vi "Manual Control - Connected Device Measurement.vi"(8 "error in":errorcluster, 10 "DER_Measurement":T1, 11 "Master Controller in":refnum<class "EMS User Interface.lvclass">) -> (0 "error out":errorcluster, 3 "Master Controller out":refnum<class "EMS User Interface.lvclass">)   [LabVIEW 2018, in "EMS User Interface Actor.lvlib" / "EMS User Interface.lvclass"]
uses:
  EMS User Interface.lvclass
  <vilib>/ORNL/CSEISMIC DDS/CSEISMIC DDS Base/Data Types/DER_Measurement.ctl
  <vilib>/ORNL/CSEISMIC DDS/CSEISMIC DDS Base/Data Types/Controls/DeviceID.ctl
  EMS User Interface.lvclass/EMS User Interface.ctl
  <vilib>/ORNL/CSEISMIC DDS/CSEISMIC DDS Base/CSEISMIC DDS.lvclass
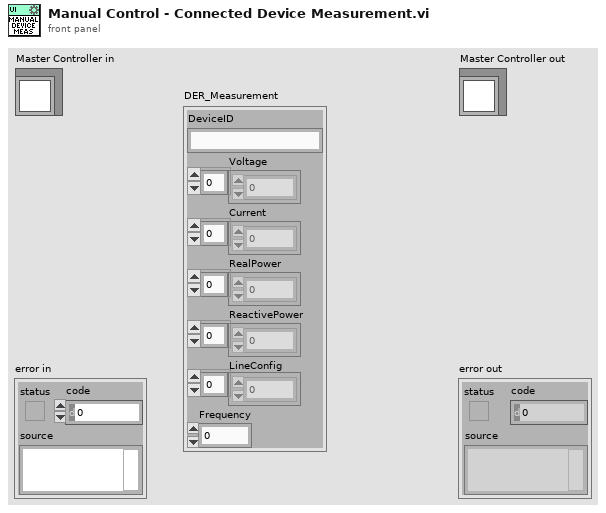
[diagram p1: front panel]
types:
  T1 = typedef "CSEISMIC DDS.lvlib/CSEISMIC DDS.lvclass/DER_Measurement.ctl" = cluster{"DeviceID":T2, "Voltage":dbl[], "Current":dbl[], "RealPower":dbl[], "ReactivePower":dbl[], "LineConfig":u8[], "Frequency":dbl}
  T2 = typedef "CSEISMIC DDS.lvlib/CSEISMIC DDS.lvclass/DeviceID.ctl" = string
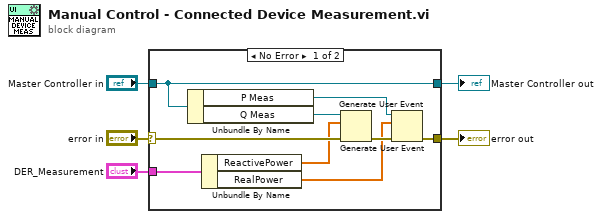
[diagram p0: block diagram]
diagram:
  n1 = case shown="No Error" "error in" {
    selector: "error in" -> [w11 w16]
    tunnel: [w10 w16] -> w4
    tunnel: [w14 w15] -> w2
    tunnel: "Master Controller in" -> [w14 w15]
    tunnel: "DER_Measurement" -> [w13 _]
    frame No Error {
      n2 = Unbundle By Name(w14) -> ("P Meas"=w8:refnum<user-event>, "Q Meas"=w9:refnum<user-event>)
      n3 = Unbundle By Name(w13) -> ("ReactivePower"=w7:dbl[], "RealPower"=w6:dbl[])
      n4 = Generate User Event(user event=w9, event data cluster=w7, error in=w11) -> (error out=w12:errorcluster)  [unwired: 1 in, 1 out]
      n5 = Generate User Event(user event=w8, event data cluster=w6, error in=w12) -> (error out=w10:errorcluster)  [unwired: 1 in, 1 out]
    }
    frame Error {
    }
  }
  "error out" <- w4
  "Master Controller out" <- w2
